vi "Call HTML Help Generation Functions Async.vi"(8 "error in (no error)":errorcluster, 9 "Extra Page Names":string[](array[string]), 11 "Destination Base Path":path) -> (0 "error out":errorcluster, 3 "Destination Base Path Out (dup)":path)   [LabVIEW 2020, in "NIVS_Consolidated_CDW_MetaDataObj.lvclass"]
doc: "Call the Copy and Create HTML file functions."
uses:
  NIVS_Consolidated_CDW_MetaDataObj.lvclass
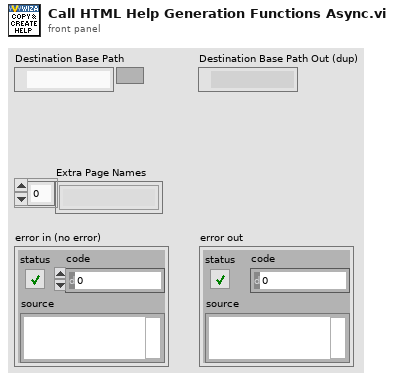
[diagram p1: front panel]
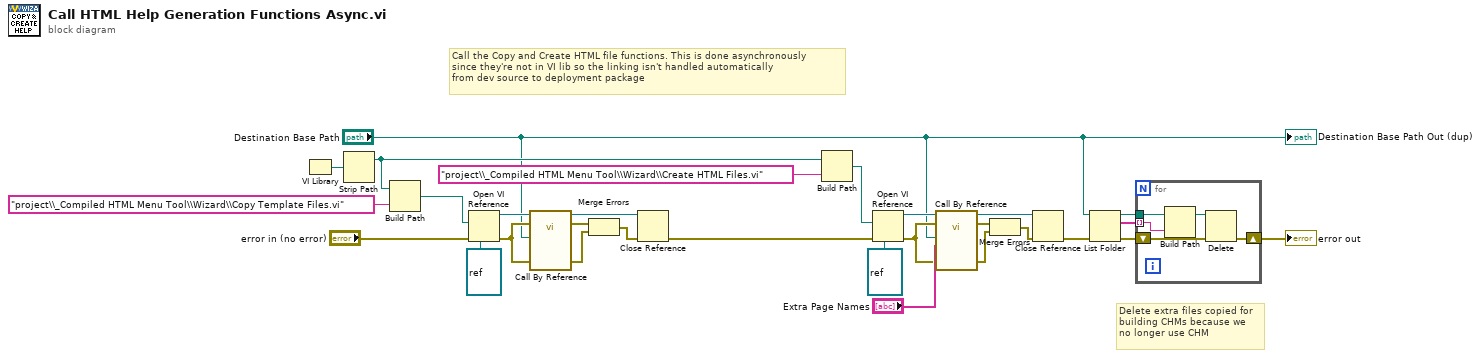
[diagram p0: block diagram]
diagram:
  # "Delete extra files copied for\nbuilding CHMs because we\nno longer use CHM"
  # "Call the Copy and Create HTML file functions. This is done asynchronously\nsince they're not in VI lib so the linking isn't handled automatically\nfrom dev source to deployment package"
  n1 = VI Library() -> (path=w7:path)
  n2 = Strip Path(path=w7) -> (stripped path=w17:path)  [unwired: 1 out]
  n3 = Build Path(base path=w17, name or relative path="project\\_Compiled HTML Menu Tool\\Wizard\\Copy Template Files.vi") -> (appended path=w9:path)
  n4 = Open VI Reference(type specifier VI Refnum (for type only)=refnum<vi> refnum, vi path=w9, error in (no error)="error in (no error)") -> (vi reference=w11:refnum<vi>, error out=w12:errorcluster)  [unwired: 3 in]
  n5 = call-by-ref "?"(reference=w11, error in=w12, 8:"error in (no error)"=w12, "Base Path"="Destination Base Path") -> (reference out=w16:refnum<vi>, error out=w13:errorcluster, 0:"error out"=w14:errorcluster)  [unwired: 9 in]
  n6 = Merge Errors(w13, w14) -> (w15:errorcluster)
  n7 = Close Reference(reference=w16, error in (no error)=w15) -> (error out=w29:errorcluster)
  n8 = Build Path(base path=w17, name or relative path="project\\_Compiled HTML Menu Tool\\Wizard\\Create HTML Files.vi") -> (appended path=w20:path)
  n9 = Open VI Reference(type specifier VI Refnum (for type only)=refnum<vi> refnum, vi path=w20, error in (no error)=w29) -> (vi reference=w22:refnum<vi>, error out=w23:errorcluster)  [unwired: 3 in]
  n10 = call-by-ref "?"(reference=w22, error in=w23, 8:"error in (no error)"=w23, "Topics"="Extra Page Names", "path"="Destination Base Path") -> (reference out=w26:refnum<vi>, error out=w27:errorcluster, 0:"error out"=w28:errorcluster)  [unwired: 8 in]
  n11 = Merge Errors(w27, w28) -> (w25:errorcluster)
  n12 = Close Reference(reference=w26, error in (no error)=w25) -> (error out=w6:errorcluster)
  n13 = List Folder(path="Destination Base Path", error in=w6) -> (path out=w4:path, filenames=w5:string[], error out=w3:errorcluster)  [unwired: 2 in, 1 out]
  n14 = for {
    tunnel: w5 -> [w33] mode=indexing
    tunnel: w4 -> [w34]
    shift-right: [w30] -> w2
    shift-left: w3 -> [w31]
    n15 = Build Path(base path=w34, name or relative path=w33) -> (appended path=w32:path)
    n16 = Delete(path (use dialog)=w32, error in=w31) -> (error out=w30:errorcluster)  [unwired: 3 in, 2 out]
  }
  "error out" <- w2
  "Destination Base Path Out (dup)" <- "Destination Base Path"
